vi "Pockels Cal-Cal explorer window.vi"() -> ()   [LabVIEW 2020]
uses:
  <vilib>/Utility/miscctls.llb/LVPointTypeDef.ctl
  Global Variables/General Globals.vi
  Configuration code/Calibration/Globals/gl_Calibration globals.vi
panel:
  out "Active file":string
  in  "Cal files listbox":i32(listbox) caption="Calibration files available"
  in  "Use cal subset":bool
  in  "Use selected file":bool
  in  "Close":bool
  in  "Tab Control":enum32{"Graph", "Table"}(tab)
  in  "Select whole curve":bool
  in  "Cal Wav listbox":i32(listbox) caption="Calibrated wavelengths in selected file"
  in  "Pockels Calibration Graph":cluster{cluster{"Value":dbl, "Value":dbl}[]}[](graph)
  out "Cal table":string[][](table) caption="Loaded calibration file's data"
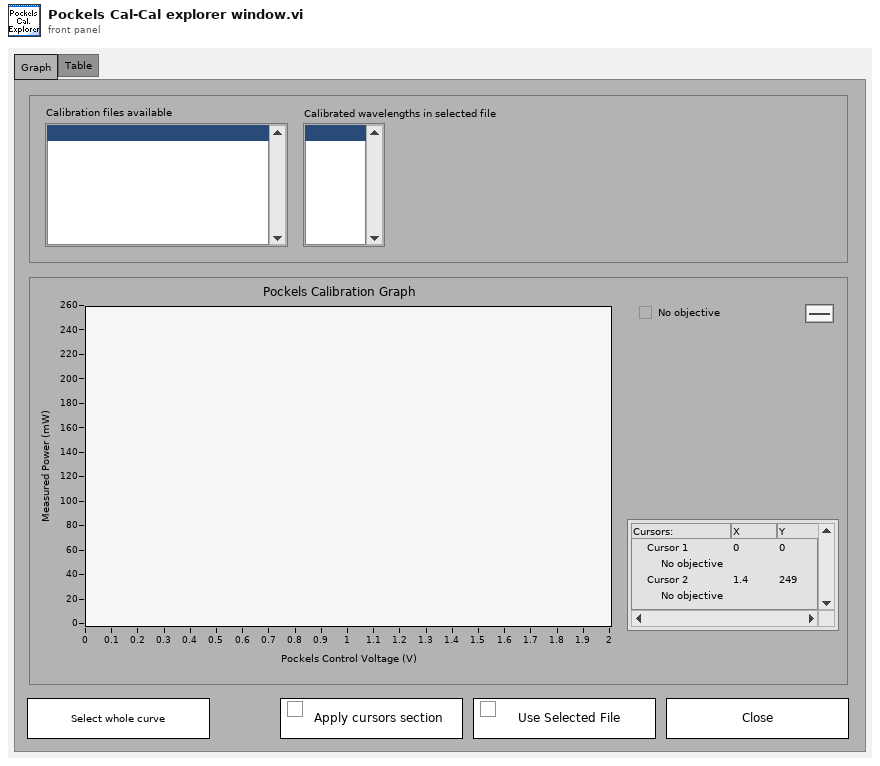
[diagram p1: front panel]
types:
  T1 = enum16{"Just read selector index", "remap to selected cal", "map to active cal"}
  T2 = typedef "LVPointTypeDef.ctl" = cluster{"Horizontal":i16, "Vertical":i16}
  T3 = enum16{"Set cursors dynamically", "Set cursors from file"}
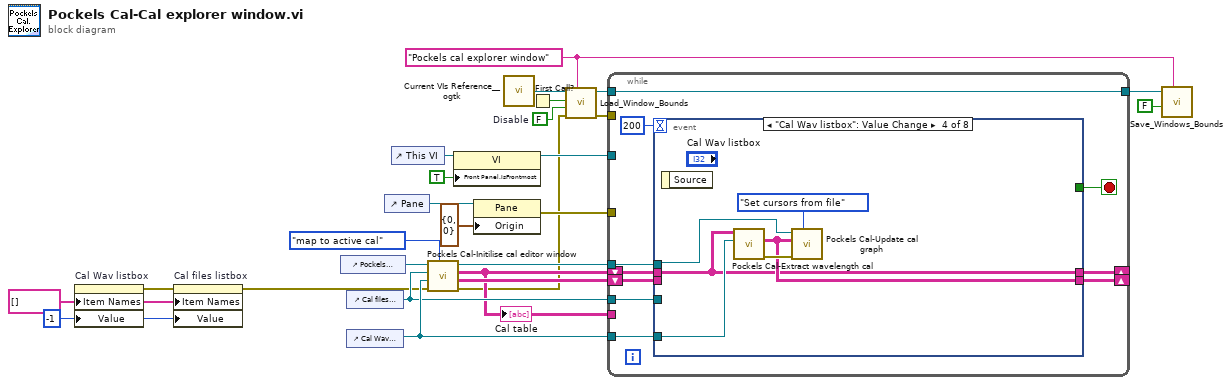
[diagram p0: block diagram]
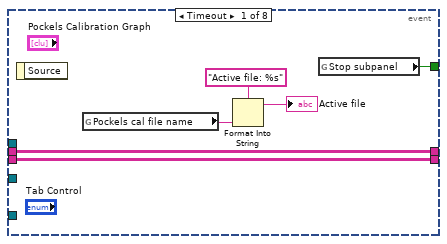
[diagram p2: hidden frame]
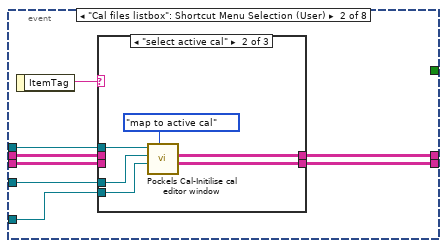
[diagram p3: hidden frame]
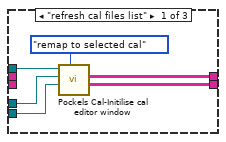
[diagram p4: hidden frame]
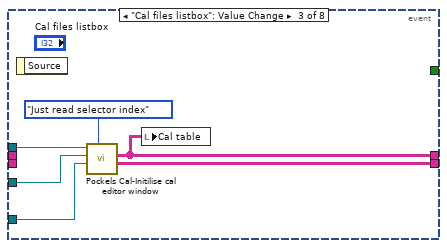
[diagram p6: hidden frame]
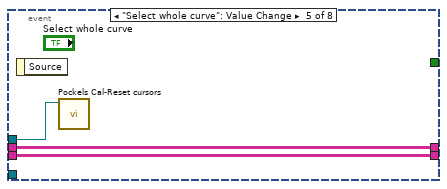
[diagram p7: hidden frame]
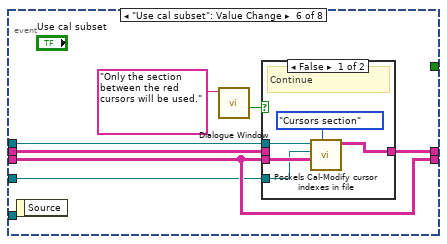
[diagram p8: hidden frame]
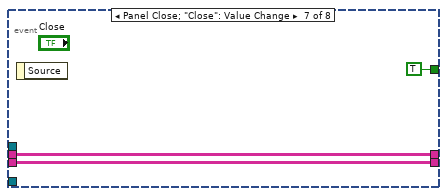
[diagram p10: hidden frame]
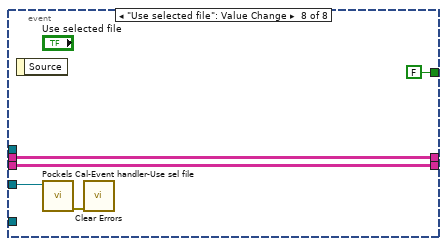
[diagram p11: hidden frame]
diagram:
  w6 = -1 ("Cal files listbox")
  w7 = string[] [] ("Item Names")
  w19 = FALSE  # Disable
  w18 = "Pockels cal explorer window" ("Window Name (i.e. Key)")
  n1 = property on="Cal Wav listbox" class="LstBox (strict)"("Item Names"=w7, "Value"=w6) -> (error out=w5:errorcluster)  [unwired: 2 in, 1 out]
  n2 = property on="Cal files listbox" class="LstBox (strict)"(error in=w5, "Item Names"=w7, "Value"=w6) -> (error out=w8:errorcluster)  [unwired: 1 in, 1 out]
  n3 = control-ref of="Pockels Calibration Graph"() -> (w13:refnum<vi>)
  n4 = control-ref of="Cal files listbox"() -> (w9:refnum<vi>)
  n5 = control-ref of="Cal Wav listbox"() -> (w11:refnum<vi>)
  n6 = control-ref of="Pane"() -> (w14:refnum<vi>)
  n7 = control-ref of="This VI"() -> (w25:refnum<vi>)
  n8 = call "Pockels Cal-Initilise cal editor window.vi"("Function"=T1."map to active cal", "error in (no error)"=w8, "Cal Wav listbox"=w11, "Cal files listbox"=w9, "XYGraph in"=w13) -> ("error out"=w2:errorcluster, "SINGLE CAL SET / Pockels Cal table (inc. headers & info)"=w10:string[][], "All data loaded"=w4:string[][], "XYGraph out"=w12:refnum<vi>)  [unwired: 3 in]
  "Cal table" <- w4
  n9 = property on="Property Node" class="VI"(reference=w25, "Front Panel.IsFrontmost"=TRUE ("Front Panel Window:Is Frontmost")) -> (reference out=w24:refnum<vi>)  [unwired: 1 in, 1 out]
  n10 = property class="Pane"(reference=w14, "Origin"=T2 {"Horizontal"=0, "Vertical"=0}) -> (error out=w22:errorcluster)  [unwired: 1 in, 1 out]
  n11 = call <userlib>:"Current VIs Reference__ogtk.vi"() -> ("Current VI's reference"=w21:refnum<vi>)  [unwired: 5 in]
  n12 = First Call?() -> (First Call?: T/F=w20:bool)
  n13 = call "Load_Window_Bounds.vi"("Window Name (i.e. Key)"=w18, "error in"=w2, "Disable"=w19, "First Call"=w20, "Window VI's Ref"=w21) -> ("error out"=w1:errorcluster, "reference out"=w16:refnum<vi>)  [unwired: 3 in, 2 out]
  n14 = while {
    tunnel: w22 -> [_]
    tunnel: w24 -> [_]
    tunnel: w16 -> [w34]
    tunnel: [w34] -> w15
    tunnel: w12 -> [w33]
    tunnel: w9 -> [w32]
    tunnel: w11 -> [w31]
    shift-right: [w30] -> _
    shift-left: w4 -> [w29]
    shift-right: [w27] -> _
    shift-left: w10 -> [w28]
    tunnel: w4 -> [_]
    tunnel: w1 -> [_]
    stop <- w36 stop-if-true
    n15 = event shown="[3] \"Cal Wav listbox\": Value Change" {
      selector: _ -> [_ _ _ _ _ _ _ _]
      dyn-events: _ -> [_ _ _ _ _ _ _ _]
      timeout: 200 -> [_ _ _ _ _ _ _ _]
      tunnel: [w42 _ _ _ _ _ TRUE ("Stop?") FALSE ("Stop?")] -> w36
      tunnel: w33 -> [_ w45 w70 w74 w78 w86 _ _]
      tunnel: w32 -> [_ w44 w69 _ _ w82 _ w98]
      tunnel: w31 -> [_ w43 w68 w75 _ _ _ _]
      tunnel: [w40 w47 w66 w71 w77 w81 w95 w96] -> w30
      tunnel: w29 -> [w40 w49 _ w71 w77 w80 w95 w96]
      tunnel: w28 -> [w41 w48 _ _ w79 w83 w94 w99]
      tunnel: [w41 w46 w67 w73 w79 w83 w94 w99] -> w27
      event Timeout {
        n16 = event-data() -> ()  [unwired: 1 in, 1 out]
        n17 = global read "gl_Calibration globals.vi" "Pockels cal file name"() -> (w37:string)
        n18 = Format Into String(format string="Active file: %s", w37) -> (resulting string=→"Active file":string)  [unwired: 2 in, 1 out]
        n19 = global read "General Globals.vi" "Stop subpanel"() -> (w42:bool)
      }
      event "Cal files listbox": Shortcut Menu Selection (User) {
        n20 = event-data() -> ("ItemTag"=w50:string)  [unwired: 1 in]
        n21 = case shown="\"select active cal\"" w50 {
          tunnel: w49 -> [_ _ w64]
          tunnel: w48 -> [_ _ w63]
          tunnel: [w56 w62 w64] -> w47
          tunnel: [w55 w61 w63] -> w46
          tunnel: w45 -> [w54 w60 _]
          tunnel: w44 -> [w53 w59 _]
          tunnel: w43 -> [w52 w58 _]
          frame "refresh cal files list" {
            n22 = call "Pockels Cal-Initilise cal editor window.vi"("Function"=T1."remap to selected cal", "Cal Wav listbox"=w52, "Cal files listbox"=w53, "XYGraph in"=w54) -> ("SINGLE CAL SET / Pockels Cal table (inc. headers & info)"=w55:string[][], "All data loaded"=w56:string[][])  [unwired: 4 in, 2 out]
          }
          frame "select active cal" {
            n23 = call "Pockels Cal-Initilise cal editor window.vi"("Function"=T1."map to active cal", "Cal Wav listbox"=w58, "Cal files listbox"=w59, "XYGraph in"=w60) -> ("SINGLE CAL SET / Pockels Cal table (inc. headers & info)"=w61:string[][], "All data loaded"=w62:string[][])  [unwired: 4 in, 2 out]
          }
          frame Default {
          }
        }
      }
      event "Cal files listbox": Value Change {
        n24 = event-data() -> ()  [unwired: 1 in, 1 out]
        n25 = call "Pockels Cal-Initilise cal editor window.vi"("Function"=T1."Just read selector index", "Cal Wav listbox"=w68, "Cal files listbox"=w69, "XYGraph in"=w70) -> ("SINGLE CAL SET / Pockels Cal table (inc. headers & info)"=w67:string[][], "All data loaded"=w66:string[][])  [unwired: 4 in, 2 out]
        n26 = local write "Cal table"(w66) -> ()
      }
      event "Cal Wav listbox": Value Change {
        n27 = event-data() -> ()  [unwired: 1 in, 1 out]
        n28 = call "Pockels Cal-Extract wavelength cal.vi"("Cal Wav listbox"=w75, "All data loaded"=w71) -> ("error IO"=w76:errorcluster, "SINGLE CAL SET / Pockels Cal table (inc. headers & info)"=w73:string[][])  [unwired: 8 in]
        n29 = call "Pockels Cal-Update cal graph.vi"("Function"=T3."Set cursors from file", "error in (no error)"=w76, "Cal table"=w73, "XYGraph in"=w74) -> ()  [unwired: 6 in, 2 out]
      }
      event "Select whole curve": Value Change {
        n30 = event-data() -> ()  [unwired: 1 in, 1 out]
        n31 = call "Pockels Cal-Reset cursors.vi"("XYGraph in"=w78) -> ()  [unwired: 9 in, 2 out]
      }
      event "Use cal subset": Value Change {
        n32 = event-data() -> ()  [unwired: 1 in, 1 out]
        n33 = call "Dialogue Window.vi"("Message string"="Only the section between the red cursors will be used.") -> ("Cancelled (Left button pressed)"=w85:bool)  [unwired: 8 in, 2 out]
        n34 = case shown="False" w85 {
          tunnel: w86 -> [w90 _]
          tunnel: w83 -> [w89 _]
          tunnel: w82 -> [w88 _]
          tunnel: [w87 w92] -> w81
          tunnel: w80 -> [_ w92]
          frame False {
            # "Continue"
            n35 = call "Pockels Cal-Modify cursor indexes in file.vi"("Function"=enum16{"Whole cal", "Cursors section"}."Cursors section", "SINGLE CAL SET / Pockels Cal table"=w89, "Cal files listbox"=w88, "XYGraph in"=w90) -> ("All data loaded"=w87:string[][])  [unwired: 7 in]
          }
          frame True {
            # "Cancelled"
          }
        }
      }
      event Panel Close; "Close": Value Change {
        n36 = event-data() -> ()  [unwired: 1 in, 1 out]
      }
      event "Use selected file": Value Change {
        n37 = event-data() -> ()  [unwired: 1 in, 1 out]
        n38 = call "Pockels Cal-Event handler-Use sel file.vi"("Cal files listbox"=w98) -> ("error out"=w97:errorcluster)  [unwired: 10 in]
        n39 = call <vilib>:"Clear Errors.vi"("error in (no error)"=w97) -> ()  [unwired: 5 in, 2 out]
      }
    }
  }
  n40 = call "Save_Windows_Bounds.vi"("Window Name (i.e. Key)"=w18, "Front Panel Window:Open"=FALSE, "Window VI's Ref"=w15) -> ()  [unwired: 8 in, 1 out]
